vi "FindTemplateMethod.vi"(10 "TemplatePath To Use first":path, 11 "TemplatePath in":path) -> (3 "TemplatePath out":path)   [LabVIEW 2020, in "ClassWriterNative.lvclass"]
uses:
  <resource>/Framework/Providers/Open_GDS/ClassProviders/Provider_LvNativeClass/ClassWriterNative_class/ClassWriterNative.lvclass
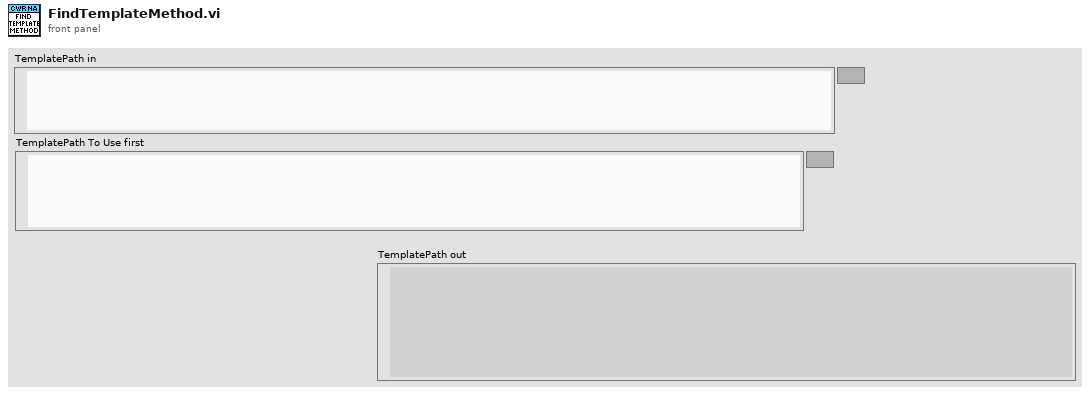
[diagram p1: front panel]
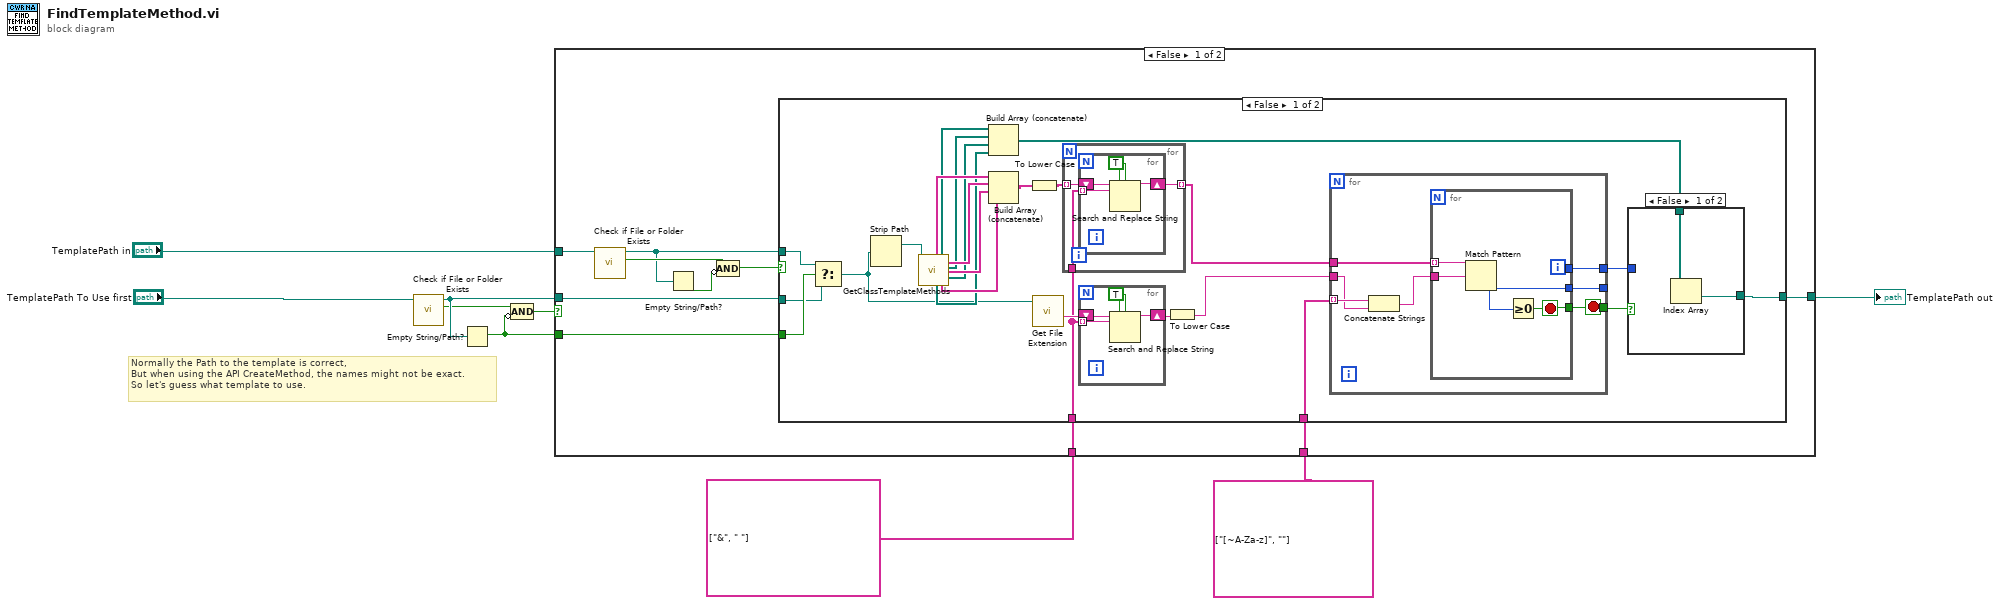
[diagram p0: block diagram]
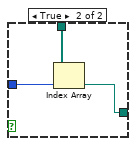
[diagram p2: hidden frame]
diagram:
  # "Normally the Path to the template is correct, \nBut when using the API CreateMethod, the names might not be exact.\nSo let's guess what template to use."
  n1 = call <vilib>:"Check if File or Folder Exists.vi"("path"="TemplatePath To Use first") -> ("file or folder exists?"=w5:bool, "dup path"=w6:path)  [unwired: 8 in, 1 out]
  n2 = Empty String/Path?(string/path=w6) -> (empty?=w1:bool)
  n3 = Compound Arithmetic op=AND(w5, invert w1) -> (w4:bool)
  n4 = case shown="False" w4 {
    tunnel: [w15 w74] -> w8
    tunnel: w6 -> [w12 w74]
    tunnel: "TemplatePath in" -> [w19 _]
    tunnel: string[] ["&", " "] -> [w14 _]
    tunnel: string[] ["[~A-Za-z]", ""] -> [w13 _]
    tunnel: w1 -> [w10 _]
    frame False {
      n5 = call <vilib>:"Check if File or Folder Exists.vi"("path"=w19) -> ("file or folder exists?"=w17:bool, "dup path"=w11:path)  [unwired: 8 in, 1 out]
      n6 = Empty String/Path?(string/path=w11) -> (empty?=w18:bool)
      n7 = Compound Arithmetic op=AND(w17, invert w18) -> (w16:bool)
      n8 = case shown="False" w16 {
        tunnel: w12 -> [w22 _]
        tunnel: [w26 w73] -> w15
        tunnel: w14 -> [w28 _]
        tunnel: w13 -> [w41 _]
        tunnel: w11 -> [w21 w73]
        tunnel: w10 -> [w23 _]
        frame False {
          n9 = Select(t=w21, s=w23, f=w22) -> (s? t:f=w20:path)
          n10 = Strip Path(path=w20) -> (stripped path=w24:path)  [unwired: 1 out]
          n11 = call <resource>:"GetClassTemplateMethods.vi"("MethodTemplatePath"=w24) -> ("NormalMethodNames"=w40:string[], "PropertyNodeMethodPaths"=w33:path[], "NormalMethodPaths"=w36:path[], "PropertyNodeMethodNames"=w37:string[], "OverrideMethodNames"=w39:string[], "OverrideMethodPaths"=w35:path[], "PropertyMethodNames"=w38:string[], "PropertyMethodPaths"=w34:path[])  [unwired: 10 in, 1 out]
          n12 = Build Array (concatenate)(w36, w35, w34, w33) -> (w30:path[])
          n13 = Build Array (concatenate)(w40, w39, w38, w37) -> (w32:string[])
          n14 = To Lower Case(string=w32) -> (all lower case string=w29:string[])
          n15 = call <vilib>:"Get File Extension.vi"("file"=w20) -> ("filename without extension"=w44:string)  [unwired: 6 in, 4 out]
          n16 = for {
            tunnel: w29 -> [w52] mode=indexing
            tunnel: w28 -> [w51]
            tunnel: [w50] -> w27 mode=indexing
            n17 = for {
              tunnel: w51 -> [w54] mode=indexing
              shift-right: [w53] -> w50
              shift-left: w52 -> [w56]
              w55 = TRUE ("replace all? (F)")
              n18 = Search and Replace String(replace all?=w55, case sensitive?=w55, input string=w56, search string=w54) -> (result string=w53:string)  [unwired: 4 in, 3 out]
            }
          }
          n19 = for {
            tunnel: w28 -> [w70] mode=indexing
            shift-right: [w69] -> w43
            shift-left: w44 -> [w72]
            w71 = TRUE ("replace all? (F)")
            n20 = Search and Replace String(replace all?=w71, case sensitive?=w71, input string=w72, search string=w70) -> (result string=w69:string)  [unwired: 4 in, 3 out]
          }
          n21 = To Lower Case(string=w43) -> (all lower case string=w42:string)
          n22 = for {
            tunnel: w27 -> [w63]
            tunnel: w42 -> [w61]
            tunnel: w41 -> [w62] mode=indexing
            tunnel: [w59] -> _
            tunnel: [w58] -> w31
            tunnel: [w57] -> w25
            stop <- w57 stop-if-true
            n23 = Concatenate Strings(w62, w61) -> (w60:string)
            n24 = for {
              tunnel: w63 -> [w68] mode=indexing
              tunnel: w60 -> [w67]
              tunnel: [w66] -> w57
              tunnel: [w65] -> w59
              tunnel: [w64] -> w58
              i -> [w64]
              stop <- w66 stop-if-true
              n25 = Match Pattern(string=w68, regular expression=w67) -> (offset past match=w65:i32)  [unwired: 1 in, 3 out]
              n26 = Greater Or Equal To 0?(x=w65) -> (x >= 0?=w66:bool)
            }
          }
          n27 = case shown="False" w25 {
            tunnel: w31 -> [_ w49]
            tunnel: w30 -> [w46 w48]
            tunnel: [w45 w47] -> w26
            frame False {
              n28 = Index Array(array=w46) -> (element=w45:path)  [unwired: 1 in]
            }
            frame True {
              n29 = Index Array(array=w48, index=w49) -> (element=w47:path)
            }
          }
        }
        frame True {
        }
      }
    }
    frame True {
    }
  }
  "TemplatePath out" <- w8
